vi "nism.zeroOrderHold.risingEdgeBool(Modified).vi"(0 "min pulse":u16, 2 "input":bool) -> (1 "output":bool)   [LabVIEW 2014]
uses:
  <vilib>/Motion/MotorControl/NI_SoftMotion_MotorControlIP.lvlib
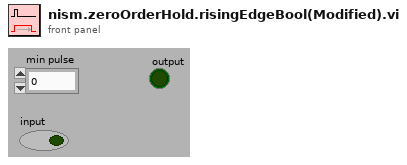
[diagram p1: front panel]
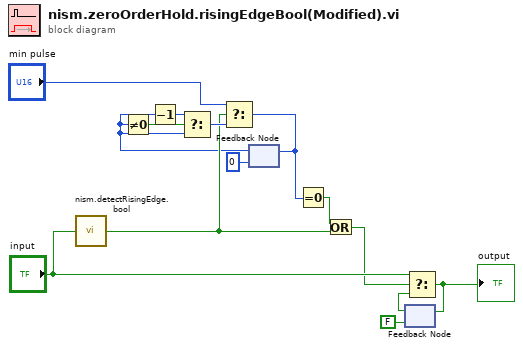
[diagram p0: block diagram]
diagram:
  n1 = call <vilib>:"nism.detectRisingEdge.bool.vi"("x"="input") -> ("y"=w6:bool)
  n2 = feedback #1(u16 0 ("min tick")) -> (w2:u16)
  n3 = Not Equal To 0?(x=w2) -> (x != 0?=w8:bool)
  n4 = Decrement(x=w2) -> (x-1=w3:u16)
  n5 = Select(t=w3, s=w8, f=w2) -> (s? t:f=w7:u16)
  n6 = Select(t="min pulse", s=w6, f=w7) -> (s? t:f=w1:u16)
  n7 = feedback-in #1(w1) -> ()
  n8 = Equal To 0?(x=w1) -> (x = 0?=w5:bool)
  n9 = Or(x=w5, y=w6) -> (x .or. y?=w4:bool)
  n10 = feedback #2(FALSE) -> (w12:bool)
  n11 = Select(t="input", s=w4, f=w12) -> (s? t:f=w14:bool)
  "output" <- w14
  n12 = feedback-in #2(w14) -> ()
